vi "Main Reversi.vi"(8 "error in (no error)":errorcluster, 9 "Wait per Turn (ms)":u32(slide) scale=0.0..1000.0, 10 "Games Per Match":u32=1 min=1 max=1000, 11 "Game Mode":T1(ring)) -> (0 "error out":errorcluster)   [LabVIEW 2020, in "Reversi.lvlib" / "Reversi.lvclass"]
uses:
  Reversi.lvclass
  Space Ring.ctl
  Reversi.lvclass/Reversi.ctl
  <vilib>/Utility/miscctls.llb/LVMapReplaceAction.ctl
  Player/Player.lvclass
panel:
  in  "Close":bool
  out "Win Count":i32(listbox)
  out "Running Stats":i32(listbox)
  out "Current Turn":T2
  in  "Stop":bool
  out "Board":T2[][](array[typedef])
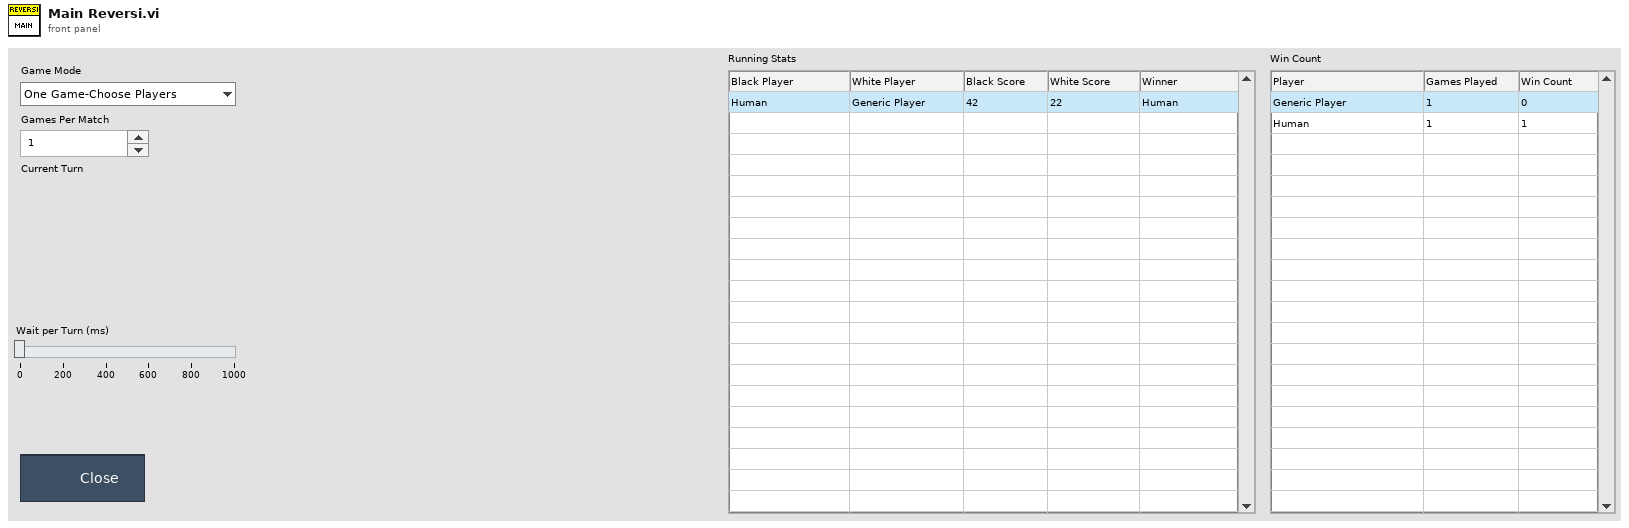
[diagram p1: front panel]
types:
  T1 = enum16{"One Game-Choose Players", "Challenge Matches (All Players)"}
  T2 = typedef "Reversi.lvlib/Reversi.lvclass/Space Ring.ctl" = u16
  T3 = cluster{"Black":refnum<class "Player.lvclass">, "White":refnum<class "Player.lvclass">}
  T4 = cluster{"Black":refnum<class "Player.lvclass">, "White":refnum<class "Player.lvclass">}[]
  T5 = cluster{"Player out":refnum<class "Player.lvclass">, "Player out":refnum<class "Player.lvclass">}
  T6 = typedef "LVMapReplaceAction.ctl" = enum32{"Modify Entry only if found", "Add or Modify Entry", "Delete Entry"}
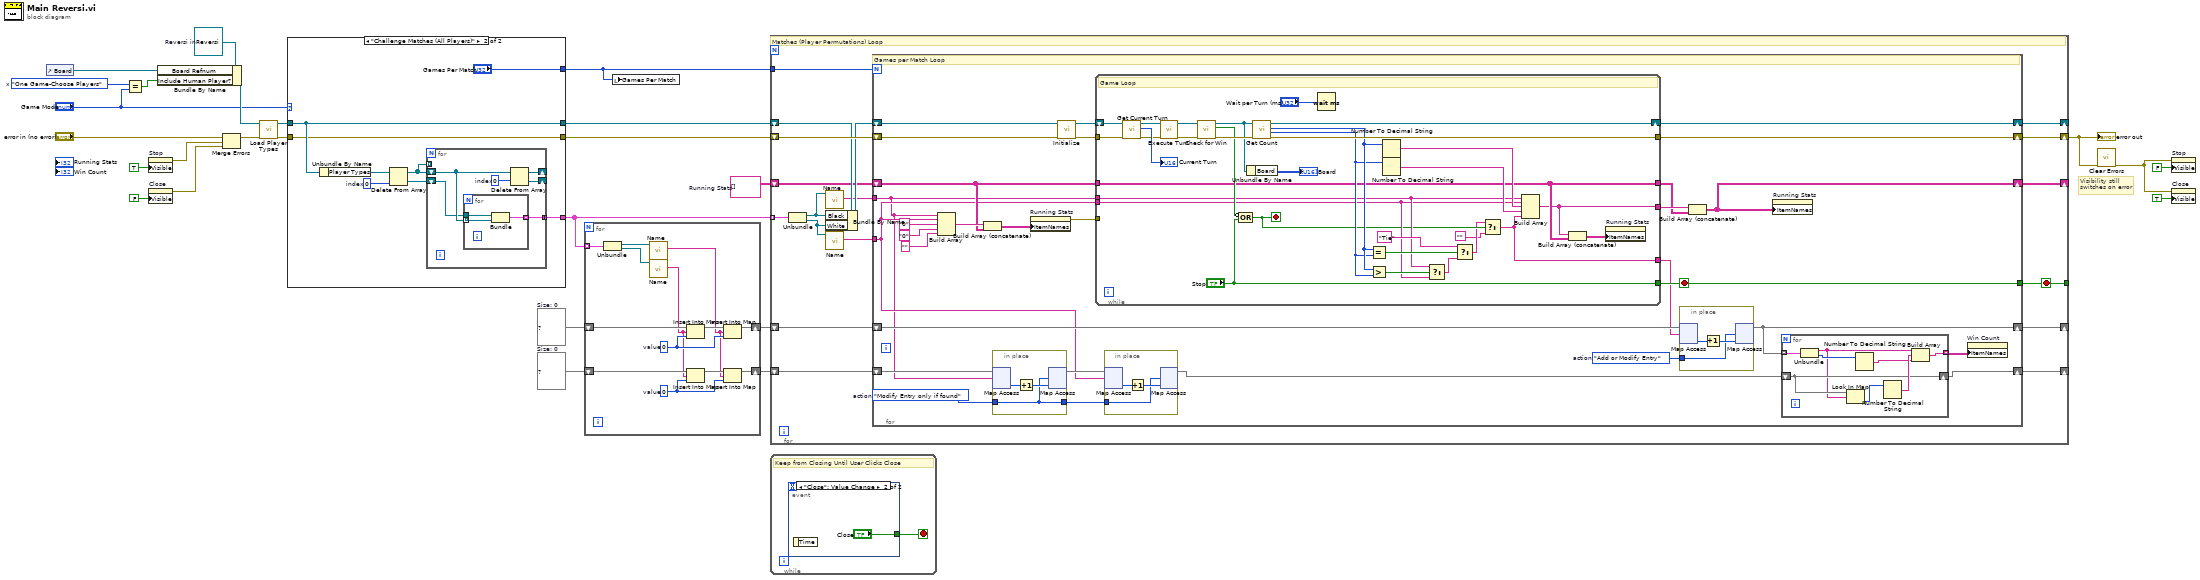
[diagram p0: block diagram]
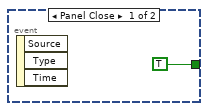
[diagram p2: hidden frame]
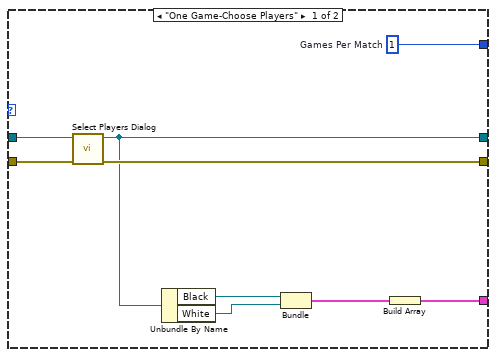
[diagram p3: hidden frame]
diagram:
  w26 = refnum<class "Reversi.lvclass"> refnum  # Reversi in
  w12 = T1."One Game-Choose Players"  # x
  w15 = map{string, i32} {}  # Size: 0
  w18 = map{string, i32} {}  # Size: 0
  w19 = string[][] []  # Running Stats
  # "Visibility still switches on error"
  n1 = control-ref of="Board"() -> (w27:refnum<vi>)
  n2 = Equal?(x=w12, y="Game Mode") -> (x = y?=w11:bool)
  n3 = property on="Stop" class="Bool"("Visible"=TRUE) -> (error out=w6:errorcluster)  [unwired: 2 in, 1 out]
  n4 = property on="Close" class="Bool"("Visible"=FALSE) -> (error out=w5:errorcluster)  [unwired: 2 in, 1 out]
  n5 = Bundle By Name(cluster=w26, "Board Refnum"=w27, "Include Human Player?"=w11) -> (w25:refnum<class "Reversi.lvclass">)
  n6 = Merge Errors("error in (no error)", w6, w5) -> (w7:errorcluster)
  n7 = call "Load Player Types.vi"("error in"=w7, "Reversi in"=w25) -> ("error out"=w22:errorcluster, "Reversi out"=w23:refnum<class "Reversi.lvclass">)  [unwired: 8 in]
  n8 = case shown="\"Challenge Matches (All Players)\"" "Game Mode" {
    tunnel: [w29 w44] -> w17
    tunnel: w23 -> [w36 w39]
    tunnel: w22 -> [w35 w38]
    tunnel: [w33 w39] -> w21
    tunnel: [w34 w38] -> w20
    tunnel: [w28 "Games Per Match"] -> w10
    frame "One Game-Choose Players" {
      w28 = u32 1  # Games Per Match
      n9 = call "Select Players Dialog.vi"("error in (no error)"=w35, "Reversi in"=w36) -> ("error out"=w34:errorcluster, "Reversi out"=w33:refnum<class "Reversi.lvclass">)  [unwired: 8 in]
      n10 = Unbundle By Name(w33) -> ("Black"=w32:refnum<class "Player.lvclass">, "White"=w31:refnum<class "Player.lvclass">)
      n11 = Bundle("Black"=w32, "White"=w31) -> (w30:T3)  [unwired: 1 in]
      n12 = Build Array(w30) -> (w29:T4)
    }
    frame "Challenge Matches (All Players)" {
      w42 = 0  # index
      n13 = Unbundle By Name(w39) -> ("Player Types"=w43:refnum<class "Player.lvclass">[])
      n14 = Delete From Array(array=w43, index=w42) -> (deleted portion=w41:refnum<class "Player.lvclass">, array with subset deleted=w40:refnum<class "Player.lvclass">[])  [unwired: 1 in]
      n15 = for {
        shift-right: [w48] -> _
        shift-left: w40 -> [w49]
        tunnel: [w50] -> w44 mode=concatenating
        shift-right: [w45] -> _
        shift-left: w41 -> [w47]
        tunnel: w40 -> [_] mode=indexing
        w46 = 0  # index
        n16 = for {
          tunnel: w47 -> [w53]
          tunnel: w49 -> [w52] mode=indexing
          tunnel: [w51] -> w50 mode=indexing
          n17 = Bundle("Player out"=w53, "Player out"=w52) -> (w51:T5)  [unwired: 1 in]
        }
        n18 = Delete From Array(array=w49, index=w46) -> (deleted portion=w45:refnum<class "Player.lvclass">, array with subset deleted=w48:refnum<class "Player.lvclass">[])  [unwired: 1 in]
      }
    }
  }
  n19 = for {
    tunnel: w17 -> [w66] mode=indexing
    shift-right: [w60] -> w16
    shift-left: w18 -> [w63]
    shift-right: [w56] -> w14
    shift-left: w15 -> [w57]
    w59 = 0  # value
    w61 = 0  # value
    n20 = Unbundle(w66) -> ("Player out"=w65:refnum<class "Player.lvclass">, "Player out"=w64:refnum<class "Player.lvclass">)
    n21 = call-dynamic "Name.vi"("Player in"=w65) -> ("Name"=w55:string)  [unwired: 8 in, 2 out]
    n22 = call-dynamic "Name.vi"("Player in"=w64) -> ("Name"=w54:string)  [unwired: 8 in, 2 out]
    n23 = Insert Into Map(map in=w63, key=w54, value=w61) -> (map out=w62:map{string, i32})  [unwired: 2 out]
    n24 = Insert Into Map(map in=w57, key=w54, value=w59) -> (map out=w58:map{string, i32})  [unwired: 2 out]
    n25 = Insert Into Map(map in=w62, key=w55, value=w61) -> (map out=w60:map{string, i32})  [unwired: 2 out]
    n26 = Insert Into Map(map in=w58, key=w55, value=w59) -> (map out=w56:map{string, i32})  [unwired: 2 out]
  }
  n27 = local write "Games Per Match"(w10) -> ()
  n28 = for {
    shift-right: [w84] -> w2
    shift-left: w20 -> [w82]
    shift-right: [w83] -> _
    shift-left: w21 -> [w79]
    tunnel: w17 -> [w80] mode=indexing
    tunnel: w10 -> [w81]
    shift-right: [w72] -> _
    shift-left: w19 -> [w73]
    shift-right: [w70] -> _
    shift-left: w16 -> [w71]
    shift-right: [w68] -> _
    shift-left: w14 -> [w69]
    tunnel: [w67] -> _
    stop <- w67 stop-if-true
    # "Matches (Player Permutations) Loop"
    n29 = Unbundle(w80) -> ("Player out"=w77:refnum<class "Player.lvclass">, "Player out"=w76:refnum<class "Player.lvclass">)
    n30 = call-dynamic "Name.vi"("Player in"=w77) -> ("Name"=w75:string)  [unwired: 8 in, 2 out]
    n31 = Bundle By Name(cluster=w79, "Black"=w77, "White"=w76) -> (w78:refnum<class "Reversi.lvclass">)
    n32 = call-dynamic "Name.vi"("Player in"=w76) -> ("Name"=w74:string)  [unwired: 8 in, 2 out]
    n33 = for {
      N: w81 -> [_]
      tunnel: [w108] -> w67
      shift-right: [w113] -> w83
      shift-left: w78 -> [w112]
      shift-right: [w114] -> w84
      shift-left: w82 -> [w110]
      tunnel: w75 -> [w85]
      tunnel: w74 -> [w88]
      shift-right: [w99] -> w72
      shift-left: w73 -> [w103]
      shift-right: [w94] -> w70
      shift-left: w71 -> [w97]
      shift-right: [w86] -> w68
      shift-left: w69 -> [w92]
      stop <- w108 stop-if-true
      w91 = LVMapReplaceAction."Modify Entry only if found"  # action
      w95 = LVMapReplaceAction."Add or Modify Entry"  # action
      # "Games per Match Loop"
      n34 = Build Array(w85, w88, "0", "0", "") -> (w104:string[])
      n35 = Build Array (concatenate)(w104, w103) -> (w102:string[][])
      n36 = in-place {
        in-place-border: w91 -> [w118]
        in-place-border: [w118] -> w89
        n37 = in-place-map #1(w92, w85) -> (w120:i32)  [unwired: 1 in, 1 out]
        n38 = Increment(x=w120) -> (x+1=w119:i32)
        n39 = in-place-map #1(w119, w118) -> (w90:map{string, i32})  [unwired: 2 out]
      }
      n40 = property on="Running Stats" class="MCListbox (strict)"("ItemNames"=w102) -> (error out=w101:errorcluster)  [unwired: 2 in, 1 out]
      n41 = call "Initialize.vi"("error in"=w110, "Reversi in"=w112) -> ("error out"=w109:errorcluster, "Reversi out"=w111:refnum<class "Reversi.lvclass">)  [unwired: 8 in]
      n42 = while {
        shift-right: [w155] -> w113
        shift-left: w111 -> [w163]
        tunnel: w109 -> [w162]
        tunnel: [w154] -> w114
        tunnel: ["Stop"] -> w108
        tunnel: w103 -> [w139]
        tunnel: w101 -> [_]
        tunnel: [w139] -> w98
        tunnel: w85 -> [w142]
        tunnel: w88 -> [w141]
        tunnel: [w137] -> w100
        tunnel: [w133] -> w96
        stop <- w136 stop-if-true
        # "Game Loop"
        n43 = call "Get Current Turn.vi"("error in (no error)"=w162, "Reversi in"=w163) -> ("error out"=w159:errorcluster, "Current Turn"=→"Current Turn":T2, "Reversi out"=w160:refnum<class "Reversi.lvclass">)  [unwired: 7 in]
        n44 = call "Execute Turn.vi"("error in"=w159, "Reversi in"=w160) -> ("error out"=w157:errorcluster, "Reversi out"=w158:refnum<class "Reversi.lvclass">)  [unwired: 8 in]
        n45 = call "Check for Win.vi"("error in (no error)"=w157, "Reversi in"=w158) -> ("error out"=w156:errorcluster, "Any Moves Left?"=w151:bool, "Reversi out"=w153:refnum<class "Reversi.lvclass">)  [unwired: 7 in]
        n46 = Compound Arithmetic op=OR(invert w151, "Stop") -> (w136:bool)
        n47 = Unbundle By Name(w153) -> ("Board"=→"Board":T2[][])
        n48 = call "Get Count.vi"("error in (no error)"=w156, "Reversi in"=w153) -> ("error out"=w154:errorcluster, "Count of White"=w144:i16, "Count of Black"=w145:i16, "Reversi out"=w155:refnum<class "Reversi.lvclass">)  [unwired: 6 in]
        n49 = Wait (ms)(milliseconds to wait="Wait per Turn (ms)") -> ()  [unwired: 1 out]
        n50 = Equal?(x=w145, y=w144) -> (x = y?=w147:bool)
        n51 = Greater?(x=w145, y=w144) -> (0:w143:bool)
        n52 = Number To Decimal String(number=w145) -> (decimal integer string=w149:string)  [unwired: 1 in]
        n53 = Number To Decimal String(number=w144) -> (decimal integer string=w148:string)  [unwired: 1 in]
        n54 = Select(t=w142, s=w143, f=w141) -> (s? t:f=w140:string)
        n55 = Select(t="Tie", s=w147, f=w140) -> (s? t:f=w135:string)
        n56 = Select(t=w135, s=w136, f="") -> (s? t:f=w133:string)
        n57 = Build Array(w142, w141, w149, w148, w133) -> (w137:string[])
        n58 = Build Array (concatenate)(w137, w139) -> (w138:string[][])
        n59 = property on="Running Stats" class="MCListbox (strict)"("ItemNames"=w138) -> ()  [unwired: 2 in, 2 out]
      }
      n60 = in-place {
        in-place-border: w89 -> [w115]
        n61 = in-place-map #2(w90, w88) -> (w117:i32)  [unwired: 1 in, 1 out]
        n62 = Increment(x=w117) -> (x+1=w116:i32)
        n63 = in-place-map #2(w116, w115) -> (w87:map{string, i32})  [unwired: 2 out]
      }
      n64 = in-place {
        in-place-border: w95 -> [w129]
        n65 = in-place-map #3(w97, w96) -> (w131:i32)  [unwired: 1 in, 1 out]
        n66 = Increment(x=w131) -> (x+1=w130:i32)
        n67 = in-place-map #3(w130, w129) -> (w94:map{string, i32})  [unwired: 2 out]
      }
      n68 = Build Array (concatenate)(w100, w98) -> (w99:string[][])
      n69 = property on="Running Stats" class="MCListbox (strict)"("ItemNames"=w99) -> ()  [unwired: 2 in, 2 out]
      n70 = for {
        tunnel: w94 -> [w128] mode=indexing
        tunnel: [w126] -> w93 mode=indexing
        shift-right: [w124] -> w86
        shift-left: w87 -> [w124]
        n71 = Unbundle(w128) -> (w122:string, w127:i32)
        n72 = Look In Map(map=w124, key=w122) -> (value=w121:i32)  [unwired: 1 in, 1 out]
        n73 = Number To Decimal String(number=w127) -> (decimal integer string=w123:string)  [unwired: 1 in]
        n74 = Number To Decimal String(number=w121) -> (decimal integer string=w125:string)  [unwired: 1 in]
        n75 = Build Array(w122, w125, w123) -> (w126:string[])
      }
      n76 = property on="Win Count" class="MCListbox (strict)"("ItemNames"=w93) -> ()  [unwired: 2 in, 2 out]
    }
  }
  "error out" <- w2
  n77 = while {
    stop <- w164 stop-if-true
    # "Keep from Closing Until User Clicks Close"
    n78 = event shown="[1] \"Close\": Value Change" {
      selector: _ -> [_ _]
      dyn-events: _ -> [_ _]
      timeout: _ -> [_ _]
      tunnel: [TRUE "Close"] -> w164
      event Panel Close {
        n79 = event-data() -> ()  [unwired: 1 in, 3 out]
      }
      event "Close": Value Change {
        n80 = event-data() -> ()  [unwired: 1 in, 1 out]
      }
    }
  }
  n81 = call <vilib>:"Clear Errors.vi"("error in (no error)"=w2) -> ("error out"=w1:errorcluster)  [unwired: 5 in, 1 out]
  n82 = property on="Stop" class="Bool"(error in=w1, "Visible"=FALSE) -> ()  [unwired: 1 in, 2 out]
  n83 = property on="Close" class="Bool"(error in=w1, "Visible"=TRUE) -> ()  [unwired: 1 in, 2 out]
